vi "FGV.vi"(8 "input":dbl, 11 "mode":enum16{"By1", "By2"}(ring)) -> (2 "output":dbl)   [LabVIEW 2017]
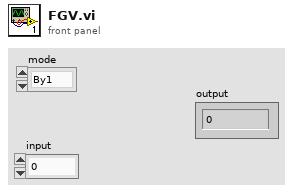
[diagram p1: front panel]
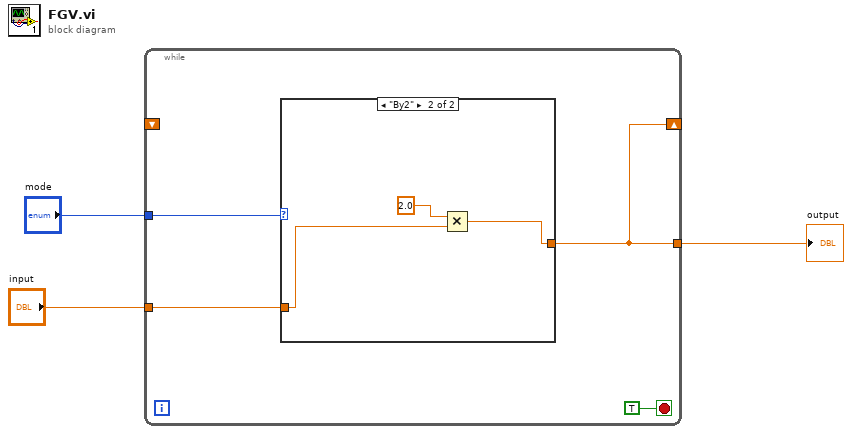
[diagram p0: block diagram]
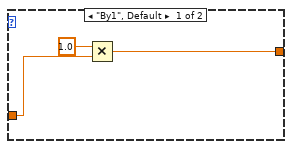
[diagram p2: hidden frame]
diagram:
  n1 = while {
    tunnel: "mode" -> [w6]
    tunnel: "input" -> [w5]
    tunnel: [w4] -> w1
    shift-right: [w4] -> _
    shift-left: _ -> [_]
    stop <- TRUE stop-if-true
    n2 = case shown="\"By2\"" w6 {
      tunnel: w5 -> [w10 w12]
      tunnel: [w8 w11] -> w4
      frame "By1", Default {
        n3 = Multiply(x=1.0, y=w10) -> (x*y=w8:dbl)
      }
      frame "By2" {
        n4 = Multiply(x=2.0, y=w12) -> (x*y=w11:dbl)
      }
    }
  }
  "output" <- w1
